vi "PH_Tektronix_7000.panel.vi"(0 "object ref":refnum<vi>, 5 "error in (no error)":errorcluster) -> (19 "error out":errorcluster)   [LabVIEW 2014, in "PH_Tektronix_7000.lvlib"]
doc: "This a GUI.\n\nLicense Agreement for this software:\n\nCopyright (C)\nGesellschaft für Schwerionenforschung, GSI\nPlanckstr. 1\n64291 Darmstadt\nGermany\n\nContact: D.Beck@gsi.de \n\nThis program is free software; you can redistribute it and/or modify it under the terms of the GNU General Public License as published by the Free Software Foundation; either version 2 of the license, or (at your option) any later version.\n\nThis program is distributed in the hope that it will be useful, but WITHOUT ANYW ARRANTY; without even the implied warranty of MERCHANTABILITY or FITNESS FOR A PARTICULAR PURPOSE. See the GNU General License for more details (http://www.gnu.org).\n\nGesellschaft für Schwerionenforschung, GSI\nPlanckstr. 1, 64291 Darmstadt, Germany\nFor all questions and ideas contact: M.Richter@gsi.de, H.Brand@gsi.de or D.Beck@gsi.de.\nLast update: 18-DEC-2002"
uses:
  PH_Tektronix_7000.lvlib
  PH_Tektronix_7000.Channel Config.ctl
  PH_Tektronix_7000.Acquisition Config.ctl
  PH_Tektronix_7000.Trigger Config.ctl
  PH_Tektronix_7000.GUI Refs.ctl
  CSCore/CSObj/CSObj.lvlib
  PH_Common/PH_Common.lvlib
  CSCore/CSSystem/CSSystemLib/CSSystemLib.lvlib
  PH_Class/PH_Class.lvlib
panel:
  out "State":u32(colorbox)
  in  "Tab Control":T1(tab)=enum."Oszilloscope Settings"
  out "Cursor: D Signal [V]":dbl format="%#p"
  out "Cursor: D Time [s]":dbl format="%#p"
  in  "Prdc Intv [ms]":i32
  in  "Save Data":bool
  in  "Fetch Data":bool
  in  "Fetch before sending Data to PSDB":bool
  out "Graph":waveform(dbl)[](graph)
  out "Data taken":timestamp
  in  "Get current Settings":bool
  in  "Name Channel 4":string
  in  "Name Channel 3":string
  in  "Name Channel 2":string
  in  "Name Channel 1":string
  in  "Allow Configure":bool
  in  "Channel 4":T2={"Enable Channel"=FALSE, "Bandwidth"=0, "Input Impedance"=0, "Vertical Coupling"=0, "Probe Attenuation"=1.0, "Range [V/div]"=1.0, "Position [div]"=10.0, "Bandwidth raw"=""} {"Vertical Coupling" items=["AC", "DC", "Ground"]; "Input Impedance" items=["1M", "50"]; "Bandwidth" items=["FULL", "500 MHz", "250 MHz", "150 MHz", "20 MHz"]}
  in  "Channel 3":T2={"Enable Channel"=FALSE, "Bandwidth"=0, "Input Impedance"=0, "Vertical Coupling"=0, "Probe Attenuation"=1.0, "Range [V/div]"=1.0, "Position [div]"=10.0, "Bandwidth raw"=""} {"Vertical Coupling" items=["AC", "DC", "Ground"]; "Input Impedance" items=["1M", "50"]; "Bandwidth" items=["FULL", "500 MHz", "250 MHz", "150 MHz", "20 MHz"]}
  in  "Trigger":T3 {"Trigger Mode" items=["Normal", "Auto"]; "Coupling" items=["DC", "AC", "Hf Reject", "Lf Reject", "Noise Rej", "Atrigger"]; "Slope" items=["Rise", "Fall", "Either"]; "Source" items=["Channel1"=0, "Channel2"=1, "Channel3"=2, "Channel4"=3, "Aux"=12, "Line"=13]}
  in  "Acquisition":T4={"Record Length"=0, "Timebase [s/div]"=10000.0, "Position [%]"=0.0, "Acquisition Type"=0, "Average Waveforms"=10, "Envelope Waveforms"=10, "WfmDB Samples"=16000, "Continuous?"=FALSE, "Delay [s]"=0.0, "Run?"=FALSE} {"Delay [s]" format="%#_12p"; "Acquisition Type" items=["Sample", "Peak Detect", "Hi Res", "Average", "Envelope", "WfmDB"]; "Timebase [s/div]" format="%#_12g"}
  in  "Channel 2":T2={"Enable Channel"=FALSE, "Bandwidth"=0, "Input Impedance"=0, "Vertical Coupling"=0, "Probe Attenuation"=1.0, "Range [V/div]"=1.0, "Position [div]"=10.0, "Bandwidth raw"=""} {"Vertical Coupling" items=["AC", "DC", "Ground"]; "Input Impedance" items=["1M", "50"]; "Bandwidth" items=["FULL", "500 MHz", "250 MHz", "150 MHz", "20 MHz"]}
  in  "Channel 1":T2={"Enable Channel"=FALSE, "Bandwidth"=0, "Input Impedance"=0, "Vertical Coupling"=0, "Probe Attenuation"=1.0, "Range [V/div]"=1.0, "Position [div]"=10.0, "Bandwidth raw"=""} {"Vertical Coupling" items=["AC", "DC", "Ground"]; "Input Impedance" items=["1M", "50"]; "Bandwidth" items=["FULL", "500 MHz", "250 MHz", "150 MHz", "20 MHz"]}
  out "Driver":string
  out "Firmware":string
  out "Serial Number":string
  out "Model":string
  out "VISA Resource":string
  out "PSDB Status":u32(colorbox)=6618880 caption="PSDB"
  in  "Delete":bool
  in  "Exit":bool
  # "PCS"
  # "3.40"
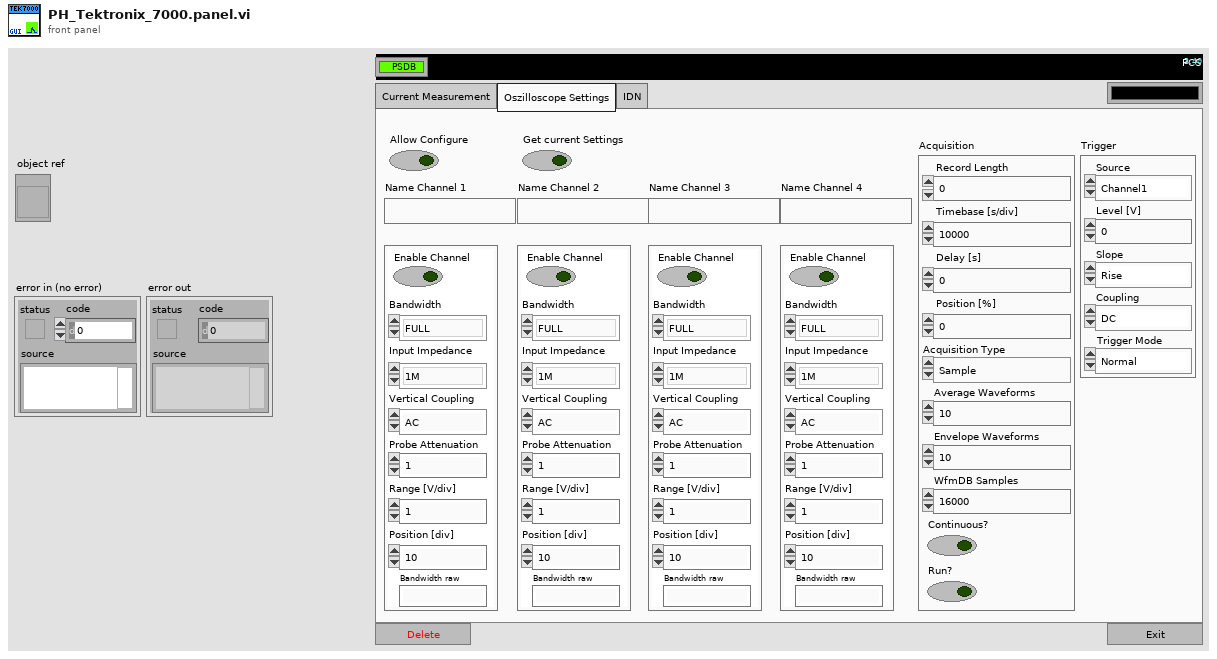
[diagram p1: front panel]
types:
  T1 = enum32{"Current Measurement", "Oszilloscope Settings", "IDN"}
  T2 = typedef "PH_Tektronix_7000.lvlib/PH_Tektronix_7000.Channel Config.ctl" = cluster{"Enable Channel":bool, "Bandwidth":u16, "Input Impedance":u16, "Vertical Coupling":u16, "Probe Attenuation":dbl, "Range [V/div]":dbl, "Position [div]":dbl, "Bandwidth raw":string}
  T3 = typedef "PH_Tektronix_7000.lvlib/PH_Tektronix_7000.Trigger Config.ctl" = cluster{"Source":u16, "Level [V]":dbl, "Slope":u16, "Coupling":u16, "Trigger Mode":u16}
  T4 = typedef "PH_Tektronix_7000.lvlib/PH_Tektronix_7000.Acquisition Config.ctl" = cluster{"Record Length":u32, "Timebase [s/div]":dbl, "Position [%]":dbl, "Acquisition Type":u16, "Average Waveforms":i32, "Envelope Waveforms":i32, "WfmDB Samples":i32, "Continuous?":bool, "Delay [s]":dbl, "Run?":bool}
  T5 = typedef "PH_Tektronix_7000.lvlib/PH_Tektronix_7000.GUI Refs.ctl" = cluster{"Graph":refnum<vi>, "State":refnum<vi>, "Delete":refnum<vi>, "VISA Resource":refnum<vi>, "Allow Configure":refnum<vi>, "Fetch Data":refnum<vi>, "Fetch before sending Data to PSDB":refnum<vi>, "Name Channel 1":refnum<vi>, "Name Channel 2":refnum<vi>, "Name Channel 3":refnum<vi>, "Name Channel 4":refnum<vi>, "Prdc Intervall [ms]":refnum<vi>, "Data taken":refnum<vi>, "Model":refnum<vi>, "Serial Number":refnum<vi>, "Firmware":refnum<vi>, "Driver":refnum<vi>, "Acquisition":refnum<vi>, "Trigger":refnum<vi>, "Cursor: D Time [s]":refnum<vi>, "Cursor: D Signal [V]":refnum<vi>, "Channel 1":refnum<vi>, "Channel 2":refnum<vi>, "Channel 3":refnum<vi>, "Channel 4":refnum<vi>}
  T6 = cluster{"TEK 7000 GUI Refs":T5, "Ref PSDB Status":refnum<vi>}
  T7 = typedef "PH_Tektronix_7000.lvlib/PH_Tektronix_7000.i attribute.ctl" = cluster{"VISA Resource Name":refnum<visa-resource-name>, "IDN":cluster{"Instrument Driver":string, "Instrument Firmware":string, "Model":string, "Serial Number":string}, "Selftest":cluster{"Result":i32, "Message":string}, "Trigger Configuration":T3, "Acquisition Configuration":T4, "GUI Refs":T5, "State":T8, "Error Message":string, "Allow Prdc Loop?":bool, "Channel 1":T2, "Channel 2":T2, "Channel 3":T2, "Channel 4":T2, "Data CH 1":waveform(dbl), "Data CH 2":waveform(dbl), "Data CH 3":waveform(dbl), "Data CH 4":waveform(dbl), "Allow config?":bool, "Name Channel 1":string, "Name Channel 2":string, "Name Channel 3":string, "Name Channel 4":string, "Fetch Data before sending to PSDB?":bool, "Constructor passed?":bool, "Data taken at":timestamp, "Plot Colors":u32[], "Default VISA Resource":string}
  T8 = typedef "PH_StatusHandler.lvlib/PH_StatusHandler.Status.ctl" = i16
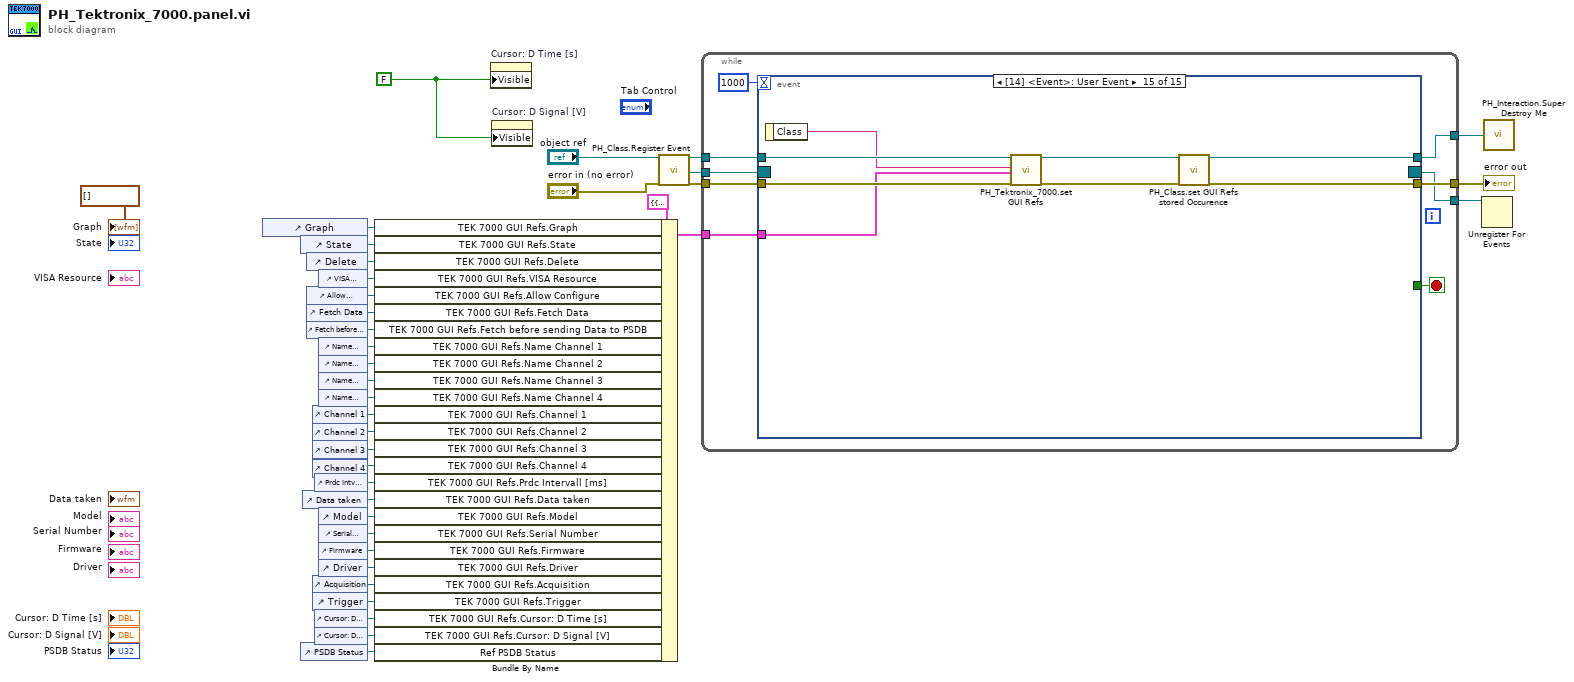
[diagram p0: block diagram]
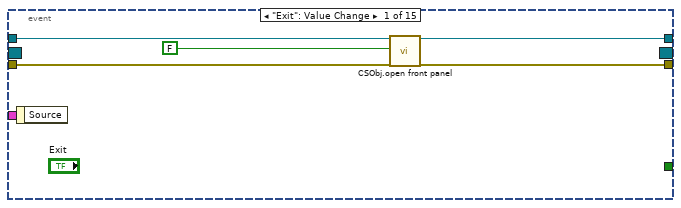
[diagram p2: hidden frame]
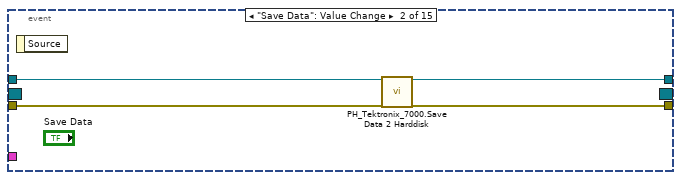
[diagram p3: hidden frame]
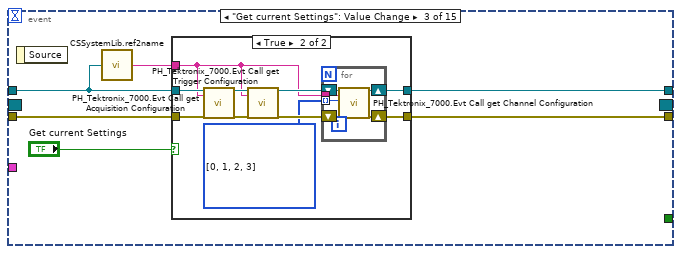
[diagram p4: hidden frame]
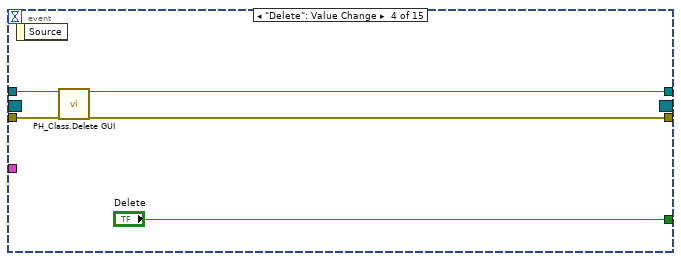
[diagram p6: hidden frame]
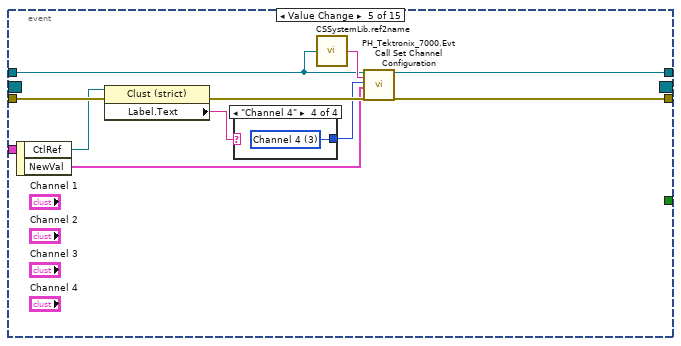
[diagram p7: hidden frame]
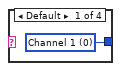
[diagram p8: hidden frame]
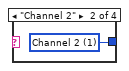
[diagram p9: hidden frame]
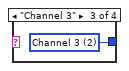
[diagram p10: hidden frame]
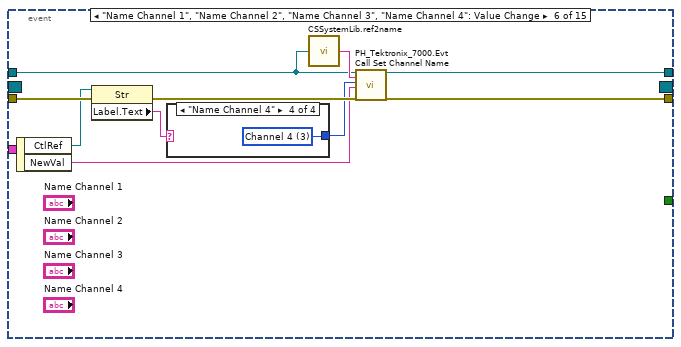
[diagram p11: hidden frame]
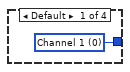
[diagram p12: hidden frame]
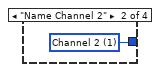
[diagram p13: hidden frame]
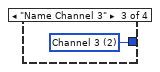
[diagram p14: hidden frame]
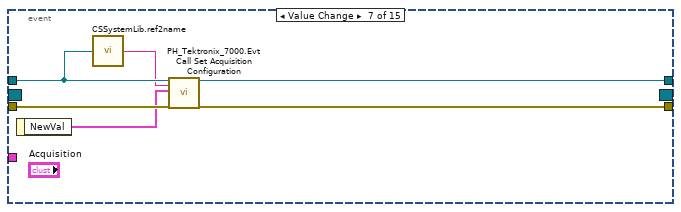
[diagram p15: hidden frame]
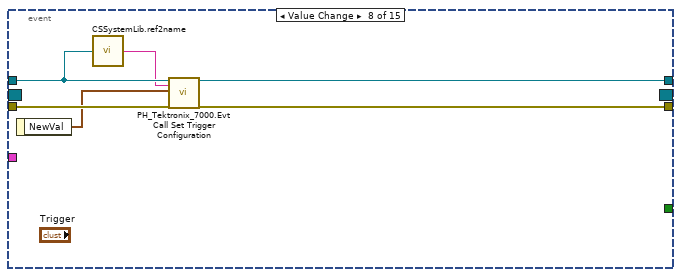
[diagram p16: hidden frame]
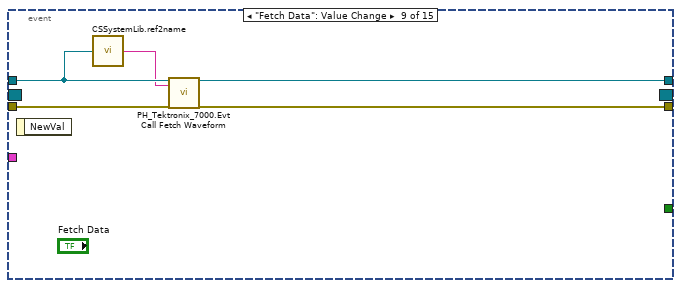
[diagram p17: hidden frame]
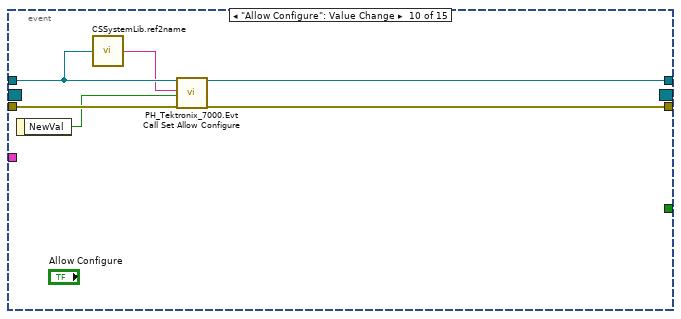
[diagram p18: hidden frame]
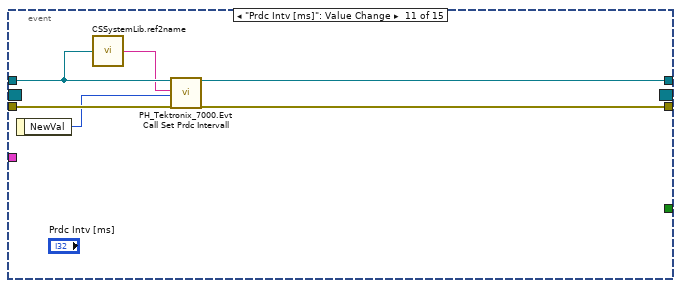
[diagram p19: hidden frame]
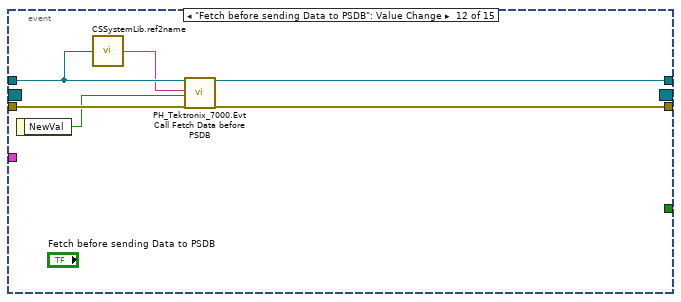
[diagram p20: hidden frame]
diagram:
  w10 = FALSE ("Visible")
  n1 = control-ref of="Graph"() -> (w35:refnum<vi>)
  n2 = control-ref of="State"() -> (w29:refnum<vi>)
  n3 = control-ref of="PSDB Status"() -> (w4:refnum<vi>)
  n4 = control-ref of="Data taken"() -> (w24:refnum<vi>)
  n5 = control-ref of="Delete"() -> (w30:refnum<vi>)
  n6 = control-ref of="Allow Configure"() -> (w13:refnum<vi>)
  n7 = control-ref of="Fetch Data"() -> (w12:refnum<vi>)
  n8 = control-ref of="Fetch before sending Data to PSDB"() -> (w11:refnum<vi>)
  n9 = control-ref of="Channel 1"() -> (w34:refnum<vi>)
  n10 = control-ref of="Channel 2"() -> (w33:refnum<vi>)
  n11 = control-ref of="Channel 3"() -> (w32:refnum<vi>)
  n12 = control-ref of="Channel 4"() -> (w31:refnum<vi>)
  n13 = control-ref of="Acquisition"() -> (w22:refnum<vi>)
  n14 = control-ref of="Trigger"() -> (w28:refnum<vi>)
  n15 = control-ref of="Prdc Intv [ms]"() -> (w25:refnum<vi>)
  n16 = control-ref of="Cursor: D Time [s]"() -> (w26:refnum<vi>)
  n17 = control-ref of="Cursor: D Signal [V]"() -> (w27:refnum<vi>)
  n18 = control-ref of="VISA Resource"() -> (w23:refnum<vi>)
  n19 = control-ref of="Name Channel 1"() -> (w14:refnum<vi>)
  n20 = control-ref of="Name Channel 2"() -> (w15:refnum<vi>)
  n21 = control-ref of="Name Channel 3"() -> (w16:refnum<vi>)
  n22 = control-ref of="Name Channel 4"() -> (w17:refnum<vi>)
  n23 = control-ref of="Model"() -> (w21:refnum<vi>)
  n24 = control-ref of="Serial Number"() -> (w20:refnum<vi>)
  n25 = control-ref of="Firmware"() -> (w19:refnum<vi>)
  n26 = control-ref of="Driver"() -> (w18:refnum<vi>)
  n27 = Bundle By Name(cluster=T6 {"TEK 7000 GUI Refs"={"Graph"=refnum, "State"=refnum, "Delete"=refnum, "VISA Resource"=refnum, "Allow Configure"=refnum, "Fetch Data"=refnum, "Fetch before sending Data to PSDB"=refnum, "Name Channel 1"=refnum, "Name Channel 2"=refnum, "Name Channel 3"=refnum, "Name Channel 4"=refnum, "Prdc Intervall [ms]"=refnum, "Data taken"=refnum, "Model"=refnum, "Serial Number"=refnum, "Firmware"=refnum, "Driver"=refnum, "Acquisition"=refnum, "Trigger"=refnum, "Cursor: D Time [s]"=refnum, "Cursor: D Signal [V]"=refnum, "Channel 1"=refnum, "Channel 2"=refnum, "Channel 3"=refnum, "Channel 4"=refnum}, "Ref PSDB Status"=refnum} ("GUI Refs"), "TEK 7000 GUI Refs.Graph"=w35, "TEK 7000 GUI Refs.State"=w29, "TEK 7000 GUI Refs.Delete"=w30, "TEK 7000 GUI Refs.VISA Resource"=w23, "TEK 7000 GUI Refs.Allow Configure"=w13, "TEK 7000 GUI Refs.Fetch Data"=w12, "TEK 7000 GUI Refs.Fetch before sending Data to PSDB"=w11, "TEK 7000 GUI Refs.Name Channel 1"=w14, "TEK 7000 GUI Refs.Name Channel 2"=w15, "TEK 7000 GUI Refs.Name Channel 3"=w16, "TEK 7000 GUI Refs.Name Channel 4"=w17, "TEK 7000 GUI Refs.Channel 1"=w34, "TEK 7000 GUI Refs.Channel 2"=w33, "TEK 7000 GUI Refs.Channel 3"=w32, "TEK 7000 GUI Refs.Channel 4"=w31, "TEK 7000 GUI Refs.Prdc Intervall [ms]"=w25, "TEK 7000 GUI Refs.Data taken"=w24, "TEK 7000 GUI Refs.Model"=w21, "TEK 7000 GUI Refs.Serial Number"=w20, "TEK 7000 GUI Refs.Firmware"=w19, "TEK 7000 GUI Refs.Driver"=w18, "TEK 7000 GUI Refs.Acquisition"=w22, "TEK 7000 GUI Refs.Trigger"=w28, "TEK 7000 GUI Refs.Cursor: D Time [s]"=w26, "TEK 7000 GUI Refs.Cursor: D Signal [V]"=w27, "Ref PSDB Status"=w4) -> (w1:T6)
  n28 = property on="Cursor: D Time [s]" class="DigNum (strict)"("Visible"=w10) -> ()  [unwired: 2 in, 2 out]
  n29 = property on="Cursor: D Signal [V]" class="DigNum (strict)"("Visible"=w10) -> ()  [unwired: 2 in, 2 out]
  n30 = call "PH_Class.Register Event.vi"("i ref in"="object ref", "error in (no error)"="error in (no error)") -> ("i ref out"=w9:refnum<vi>, "Event Registration Refnum"=w7:refnum<event-registration>, "error out"=w8:errorcluster)  [unwired: 15 in]
  n31 = while {
    tunnel: w9 -> [w44]
    tunnel: [w43] -> w38
    tunnel: w8 -> [w46]
    tunnel: [w45] -> w37
    tunnel: w7 -> [w41]
    tunnel: [w40] -> w6
    tunnel: w1 -> [w39]
    stop <- w47 stop-if-true
    n32 = event shown="[14] <Event>: User Event" {
      selector: w41 -> [_ _ _ _ _ _ _ _ _ _ _ _ _ _ _]
      dyn-events: [_ _ _ _ _ _ _ _ _ _ _ _ _ _ _] -> w40
      timeout: 1000 -> [_ _ _ _ _ _ _ _ _ _ _ _ _ _ _]
      tunnel: [_ _ _ "Delete" _ _ _ _ _ _ _ _ _ _ _] -> w47
      tunnel: w44 -> [w49 w54 w58 w84 w91 w105 w116 w122 w127 w133 w139 w145 w153 w197 w206]
      tunnel: w46 -> [w52 w55 w61 w83 w93 w107 w119 w125 w130 w136 w142 w148 w157 w198 w205]
      tunnel: [w51 w56 w62 w81 w92 w106 w118 w124 w129 w135 w141 w147 w156 w195 w200] -> w45
      tunnel: [w48 w53 w60 w82 w90 w104 w117 w123 w128 w134 w140 w146 w158 w196 w202] -> w43
      tunnel: w39 -> [_ _ _ _ _ _ _ _ _ _ _ _ _ _ w199]
      event "Exit": Value Change {
        n33 = event-data() -> ()  [unwired: 1 in, 1 out]
        n34 = call "CSObj.open front panel.vi"("i ref in"=w49, "frontPanelOpen"=FALSE ("front panel open"), "error in (no error)"=w52) -> ("i ref out"=w48:refnum<vi>, "error out"=w51:errorcluster)  [unwired: 15 in]
      }
      event "Save Data": Value Change {
        n35 = event-data() -> ()  [unwired: 1 in, 1 out]
        n36 = call "PH_Tektronix_7000.Save Data 2 Harddisk.vi"("i ref in"=w54, "error in"=w55) -> ("i ref out"=w53:refnum<vi>, "error out"=w56:errorcluster)  [unwired: 16 in]
      }
      event "Get current Settings": Value Change {
        n37 = event-data() -> ()  [unwired: 1 in, 1 out]
        n38 = call "CSSystemLib.ref2name.vi"("obj refnum"=w58) -> ("name"=w57:string)
        n39 = case shown="True" "Get current Settings" {
          tunnel: [w63 w67] -> w62
          tunnel: w61 -> [w63 w74]
          tunnel: w58 -> [w64 w73]
          tunnel: [w64 w70] -> w60
          tunnel: w57 -> [_ w66]
          frame False {
          }
          frame True {
            w65 = u16[] [0, 1, 2, 3] items=["Channel 1", "Channel 2", "Channel 3", "Channel 4", "Math 1", "Math 2", "Math 3", "Math 4", "Reference 1", "Reference 2", "Reference 3", "Reference 4"]
            n40 = call "PH_Tektronix_7000.Evt Call get Acquisition Configuration.vi"("i ref in"=w73, "Instance"=w66, "error in (no error)"=w74) -> ("i ref out"=w72:refnum<vi>, "error out"=w69:errorcluster)  [unwired: 15 in]
            n41 = call "PH_Tektronix_7000.Evt Call get Trigger Configuration.vi"("i ref in"=w72, "Instance"=w66, "error in (no error)"=w69) -> ("i ref out"=w71:refnum<vi>, "error out"=w68:errorcluster)  [unwired: 15 in]
            n42 = for {
              tunnel: w66 -> [w76]
              shift-right: [w79] -> w70
              shift-left: w71 -> [w80]
              shift-right: [w77] -> w67
              shift-left: w68 -> [w78]
              tunnel: w65 -> [w75] mode=indexing
              n43 = call "PH_Tektronix_7000.Evt Call get Channel Configuration.vi"("i ref in"=w80, "Instance"=w76, "Channel"=w75, "error in (no error)"=w78) -> ("i ref out"=w79:refnum<vi>, "error out"=w77:errorcluster)  [unwired: 14 in]
            }
          }
        }
      }
      event "Delete": Value Change {
        n44 = event-data() -> ()  [unwired: 1 in, 1 out]
        n45 = call "PH_Class.Delete GUI.vi"("VI in"=w84, "error in (no error)"=w83) -> ("VI out"=w82:refnum<vi>, "error out"=w81:errorcluster)  [unwired: 16 in]
      }
      event Value Change {
        n46 = event-data() -> ("CtlRef"=w89:refnum<vi>, "NewVal"=w88:T2)  [unwired: 1 in]
        n47 = property class="Clust (strict)"(reference=w89, error in=w93) -> (error out=w94:errorcluster, "Label.Text"=w87:string)  [unwired: 1 out]
        n48 = case shown="\"Channel 4\"" w87 {
          tunnel: [w96 w97 w98 w99] -> w86
          frame Default {
            w96 = u16 0 items=["Channel 1", "Channel 2", "Channel 3", "Channel 4", "Math 1", "Math 2", "Math 3", "Math 4", "Reference 1", "Reference 2", "Reference 3", "Reference 4"] ("Channel")
          }
          frame "Channel 2" {
            w97 = u16 1 items=["Channel 1", "Channel 2", "Channel 3", "Channel 4", "Math 1", "Math 2", "Math 3", "Math 4", "Reference 1", "Reference 2", "Reference 3", "Reference 4"] ("Channel")
          }
          frame "Channel 3" {
            w98 = u16 2 items=["Channel 1", "Channel 2", "Channel 3", "Channel 4", "Math 1", "Math 2", "Math 3", "Math 4", "Reference 1", "Reference 2", "Reference 3", "Reference 4"] ("Channel")
          }
          frame "Channel 4" {
            w99 = u16 3 items=["Channel 1", "Channel 2", "Channel 3", "Channel 4", "Math 1", "Math 2", "Math 3", "Math 4", "Reference 1", "Reference 2", "Reference 3", "Reference 4"] ("Channel")
          }
        }
        n49 = call "CSSystemLib.ref2name.vi"("obj refnum"=w91) -> ("name"=w95:string)
        n50 = call "PH_Tektronix_7000.Evt Call Set Channel Configuration.vi"("i ref in"=w91, "Instance"=w95, "Channel"=w86, "Channel Configuration"=w88, "error in (no error)"=w94) -> ("i ref out"=w90:refnum<vi>, "error out"=w92:errorcluster)  [unwired: 13 in]
      }
      event "Name Channel 1", "Name Channel 2", "Name Channel 3", "Name Channel 4": Value Change {
        n51 = event-data() -> ("CtlRef"=w103:refnum<vi>, "NewVal"=w100:string)  [unwired: 1 in]
        n52 = property class="Str"(reference=w103, error in=w107) -> (error out=w108:errorcluster, "Label.Text"=w102:string)  [unwired: 1 out]
        n53 = case shown="\"Name Channel 4\"" w102 {
          tunnel: [w110 w111 w112 w113] -> w101
          frame Default {
            w110 = u16 0 items=["Channel 1", "Channel 2", "Channel 3", "Channel 4", "Math 1", "Math 2", "Math 3", "Math 4", "Reference 1", "Reference 2", "Reference 3", "Reference 4"] ("Channel")
          }
          frame "Name Channel 2" {
            w111 = u16 1 items=["Channel 1", "Channel 2", "Channel 3", "Channel 4", "Math 1", "Math 2", "Math 3", "Math 4", "Reference 1", "Reference 2", "Reference 3", "Reference 4"] ("Channel")
          }
          frame "Name Channel 3" {
            w112 = u16 2 items=["Channel 1", "Channel 2", "Channel 3", "Channel 4", "Math 1", "Math 2", "Math 3", "Math 4", "Reference 1", "Reference 2", "Reference 3", "Reference 4"] ("Channel")
          }
          frame "Name Channel 4" {
            w113 = u16 3 items=["Channel 1", "Channel 2", "Channel 3", "Channel 4", "Math 1", "Math 2", "Math 3", "Math 4", "Reference 1", "Reference 2", "Reference 3", "Reference 4"] ("Channel")
          }
        }
        n54 = call "CSSystemLib.ref2name.vi"("obj refnum"=w105) -> ("name"=w109:string)
        n55 = call "PH_Tektronix_7000.Evt Call Set Channel Name.vi"("i ref in"=w105, "Instance"=w109, "Channel"=w101, "Channel Name"=w100, "error in (no error)"=w108) -> ("i ref out"=w104:refnum<vi>, "error out"=w106:errorcluster)  [unwired: 13 in]
      }
      event Value Change {
        n56 = event-data() -> ("NewVal"=w114:T4)  [unwired: 1 in]
        n57 = call "CSSystemLib.ref2name.vi"("obj refnum"=w116) -> ("name"=w115:string)
        n58 = call "PH_Tektronix_7000.Evt Call Set Acquisition Configuration.vi"("i ref in"=w116, "Instance"=w115, "Acquisition Configuration"=w114, "error in (no error)"=w119) -> ("i ref out"=w117:refnum<vi>, "error out"=w118:errorcluster)  [unwired: 14 in]
      }
      event Value Change {
        n59 = event-data() -> ("NewVal"=w120:T3)  [unwired: 1 in]
        n60 = call "CSSystemLib.ref2name.vi"("obj refnum"=w122) -> ("name"=w121:string)
        n61 = call "PH_Tektronix_7000.Evt Call Set Trigger Configuration.vi"("i ref in"=w122, "Instance"=w121, "Trigger Configuration"=w120, "error in (no error)"=w125) -> ("i ref out"=w123:refnum<vi>, "error out"=w124:errorcluster)  [unwired: 14 in]
      }
      event "Fetch Data": Value Change {
        n62 = event-data() -> ()  [unwired: 1 in, 1 out]
        n63 = call "CSSystemLib.ref2name.vi"("obj refnum"=w127) -> ("name"=w126:string)
        n64 = call "PH_Tektronix_7000.Evt Call Fetch Waveform.vi"("i ref in"=w127, "Instance"=w126, "error in (no error)"=w130) -> ("i ref out"=w128:refnum<vi>, "error out"=w129:errorcluster)  [unwired: 15 in]
      }
      event "Allow Configure": Value Change {
        n65 = event-data() -> ("NewVal"=w131:bool)  [unwired: 1 in]
        n66 = call "CSSystemLib.ref2name.vi"("obj refnum"=w133) -> ("name"=w132:string)
        n67 = call "PH_Tektronix_7000.Evt Call Set Allow Configure.vi"("i ref in"=w133, "Instance"=w132, "Configure allowed?"=w131, "error in (no error)"=w136) -> ("i ref out"=w134:refnum<vi>, "error out"=w135:errorcluster)  [unwired: 14 in]
      }
      event "Prdc Intv [ms]": Value Change {
        n68 = event-data() -> ("NewVal"=w137:i32)  [unwired: 1 in]
        n69 = call "CSSystemLib.ref2name.vi"("obj refnum"=w139) -> ("name"=w138:string)
        n70 = call "PH_Tektronix_7000.Evt Call Set Prdc Intervall.vi"("i ref in"=w139, "Instance"=w138, "Prc Intervall [ms]"=w137, "error in (no error)"=w142) -> ("i ref out"=w140:refnum<vi>, "error out"=w141:errorcluster)  [unwired: 14 in]
      }
      event "Fetch before sending Data to PSDB": Value Change {
        n71 = event-data() -> ("NewVal"=w143:bool)  [unwired: 1 in]
        n72 = call "CSSystemLib.ref2name.vi"("obj refnum"=w145) -> ("name"=w144:string)
        n73 = call "PH_Tektronix_7000.Evt Call Fetch Data before PSDB.vi"("i ref in"=w145, "Instance"=w144, "Fetch before PSDB?"=w143, "error in (no error)"=w148) -> ("i ref out"=w146:refnum<vi>, "error out"=w147:errorcluster)  [unwired: 14 in]
      }
      event "Graph": Plot Attribute Change {
        n74 = event-data() -> ()  [unwired: 1 in, 1 out]
        n75 = call "PH_Tektronix_7000.get data to modify.vi"("i ref in"=w153, "error in (no error)"=w157) -> ("i ref out"=w152:refnum<vi>, "i attribute"=w149:T7, "timed out"=w150:bool, "error out"=w155:errorcluster)  [unwired: 14 in]
        n76 = case shown="False" w150 {
          tunnel: w155 -> [w167 w193]
          tunnel: [w166 w193] -> w154
          tunnel: w152 -> [w165 w194]
          tunnel: [w164 w194] -> w151
          tunnel: w149 -> [w163 _]
          frame False {
            n77 = Unbundle By Name(w163) -> ("GUI Refs.Graph"=w161:refnum<vi>, "Plot Colors"=w160:u32[])
            n78 = while {
              tunnel: w161 -> [w180]
              shift-right: [w171] -> w159
              shift-left: w160 -> [w170]
              i -> [w177]
              stop <- w173 stop-if-true
              n79 = To Unsigned Long Integer(number=w177) -> (unsigned 32bit integer=w179:u32)
              n80 = property class="WFGraph (strict)"(reference=w180, "Active Plot"=w179) -> (error out=w178:errorcluster, "Plot.Plot Color"=w168:u32, "Plot.Plot Name"=w169:string)  [unwired: 1 in, 1 out]
              n81 = Equal?(x=w177, y=3) -> (x = y?=w175:bool)
              n82 = for {
                tunnel: w169 -> [w187]
                tunnel: string[] ["Channel 1", "Channel 2", "Channel 3", "Channel 4"] -> [w182] mode=indexing
                tunnel: w168 -> [w185]
                shift-right: [w184] -> w171
                shift-left: w170 -> [w186]
                i -> [w181]
                n83 = Match Pattern(string=w187, regular expression=w182) -> (offset past match=w183:i32)  [unwired: 1 in, 3 out]
                n84 = case shown="Default" w183 {
                  tunnel: w186 -> [w188 w192]
                  tunnel: w181 -> [_ w191]
                  tunnel: w185 -> [_ w190]
                  tunnel: [w188 w189] -> w184
                  frame -1 {
                  }
                  frame Default {
                    n85 = Replace Array Subset(array=w192, new element=w190, index=w191) -> (w189:u32[])
                  }
                }
              }
              n86 = Unbundle By Name(w178) -> ("status"=w174:bool)
              n87 = Or(x=w175, y=w174) -> (x .or. y?=w173:bool)
            }
            n88 = Bundle By Name(cluster=w163, "Plot Colors"=w159) -> (w162:T7)
            n89 = call "PH_Tektronix_7000.set modified data.vi"("i ref in"=w165, "i attribute"=w162, "error in (no error)"=w167) -> ("i ref out"=w164:refnum<vi>, "error out"=w166:errorcluster)  [unwired: 15 in]
          }
          frame True {
          }
        }
        n90 = call "PH_Tektronix_7000.Set Channel Name BG Color.vi"("i ref in"=w151, "error in"=w154) -> ("i ref out"=w158:refnum<vi>, "error out"=w156:errorcluster)  [unwired: 16 in]
      }
      event Timeout {
        n91 = event-data() -> ()  [unwired: 1 in, 1 out]
        n92 = call "PH_Tektronix_7000.set Cursor Deltas.vi"("i ref in"=w197, "error in (no eror)"=w198) -> ("i ref out"=w196:refnum<vi>, "error out"=w195:errorcluster)  [unwired: 16 in]
      }
      event User Event {
        n93 = event-data() -> ("Class"=w204:string)  [unwired: 1 in]
        n94 = call "PH_Tektronix_7000.set GUI Refs.vi"("i ref in"=w206, "Class"=w204, "GUI Refs"=w199, "error in (no error)"=w205) -> ("i ref out"=w203:refnum<vi>, "error out"=w201:errorcluster)  [unwired: 14 in]
        n95 = call "PH_Class.set GUI Refs stored Occurence.vi"("i ref in"=w203, "error in (no error)"=w201) -> ("i ref out"=w202:refnum<vi>, "error out"=w200:errorcluster)  [unwired: 16 in]
      }
    }
  }
  "error out" <- w37
  n96 = Unregister For Events(event registration refnum=w6) -> ()  [unwired: 1 in, 1 out]
  n97 = call "PH_Interaction.Super Destroy Me.vi"("i ref out"=w38) -> ()
  "Graph" <- waveform(dbl)[] [] ("Graph")
